vi "Switch status IO - Human Readable.vi"(1 "Switch status":path=path "C:/LabView/PPMS basic VIs/Switch Status.txt") -> (0 "String":string)   [LabVIEW 2011]
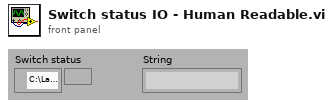
[diagram p1: front panel]
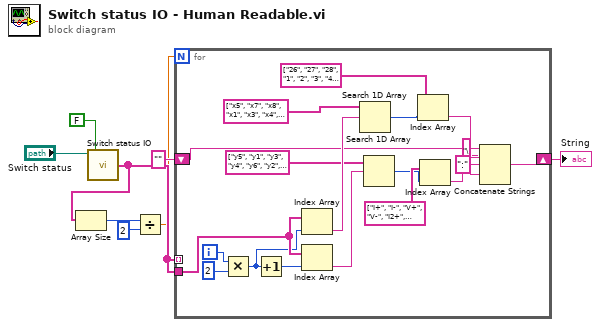
[diagram p0: block diagram]
diagram:
  n1 = call "Switch status IO.vi"("Write: T\nRead: F"=FALSE ("Write: T\nRead: F"), "Path"="Switch status") -> ("String out"=w6:string[])  [unwired: 4 in]
  n2 = Array Size(array=w6) -> (size(s)=w3:i32)
  n3 = Divide(x=w3, y=2) -> (x/y=w5:dbl)
  n4 = for {
    N: w5 -> [_]
    tunnel: w6 -> [w27]
    tunnel: w6 -> [_] mode=indexing
    shift-right: [w14] -> w8
    shift-left: "" -> [w13]
    i -> [w25]
    n5 = Multiply(x=w25, y=2) -> (x*y=w23:i32)
    n6 = Increment(x=w23) -> (x+1=w26:i32)
    n7 = Index Array(array=w27, index=w23) -> (element=w21:string)
    n8 = Index Array(array=w27, index=w26) -> (element=w17:string)
    n9 = Search 1D Array(1D array=string[] ["x5", "x7", "x8", "x1", "x3", "x4", "x2", "x6"], element=w21) -> (index of element=w19:i32)  [unwired: 1 in]
    n10 = Search 1D Array(1D array=string[] ["y5", "y1", "y3", "y4", "y6", "y2", "y7", "y8"], element=w17) -> (index of element=w15:i32)  [unwired: 1 in]
    n11 = Index Array(array=string[] ["26", "27", "28", "1", "2", "3", "4", "5"], index=w19) -> (element=w10:string)
    n12 = Index Array(array=string[] ["I+", "I-", "V+", "V-", "I2+", "I2-", "V2+", "V2-"], index=w15) -> (element=w12:string)
    n13 = Concatenate Strings(w13, w12, ":" ("string"), w10, "\n" ("string")) -> (w14:string)
  }
  "String" <- w8
